vi "Actor Core.vi"(0 "Module in":refnum<class "Module.lvclass">, 11 "Error in":errorcluster caption="Error in (no error)") -> (4 "Module out":refnum<class "Module.lvclass">, 15 "Error out":errorcluster)   [LabVIEW 2019, in "GP Module.lvlib" / "Module.lvclass"]
doc: "GPower Actor Core VI.\n\nSteen Schmidt\nGPower\n9/9 2018"
uses:
  Module.lvclass
  C:/Program Files (x86)/National Instruments/LabVIEW 2019/vi.lib/GPower/Actor/Library/Actor Class/Actor.lvclass
  Module.lvclass/Module.ctl
  <vilib>/GPower/Actor/Library/Actor Class/Actor.lvclass/Actor.ctl
  <vilib>/GPower/Actor/Library/Actor Interface Class/Actor Interface.lvclass/Actor Interface.ctl
  <vilib>/GPower/Message/Library/Message Class/Message.lvclass/Message.ctl
  <vilib>/GPower/Logger/Library/Logger Class/Logger.lvclass/Logger.ctl
  <vilib>/GPower/Actor/Library/Actor Interface Class/Accessors/Get Actor Name.vi
  <vilib>/GPower/Logger/Library/Logger Class/Logger/Log.vi
  <vilib>/GPower/Message/Library/Message Class/Accessors/Get Name.vi
  <vilib>/GPower/Error/Library/ErrorType.vi
  <vilib>/GPower/Logger/Library/Logger Class/Accessors/Get Enabled State.vi
  <vilib>/GPower/Logger/Library/Logger Class/Accessors/Get Severity Level Threshold.vi
  <vilib>/GPower/Logger/Library/Logger Class/Logger/Promote.vi
  <vilib>/GPower/Error/Library/SplitAppended.vi
  <vilib>/GPower/Logger/Library/Logger Class/Accessors/Get Error And Warning Promotion.vi
  <vilib>/GPower/Error/Library/SubVIs/ExplanationToError.vi
  <vilib>/dlg_ctls.llb/Space Constant.vi
  <vilib>/Utility/error.llb/Trim Whitespace.vi
  <vilib>/Utility/error.llb/Error Code Database.vi
  <vilib>/GPower/Error/Library/SubVIs/SetStatus.vi
  <vilib>/GPower/Error/Library/AppendErrors.vi
  <vilib>/GPower/Error/Library/Append/AppendSingle.vi
  <vilib>/GPower/Logger/Library/Logger Class/Logger.lvclass
  <vilib>/GPower/Actor/Library/Actor Class/Actor.lvclass
  <vilib>/GPower/Actor/Library/Responder Class/Responder.lvclass
panel:
  in  "Stop":bool
  out "Boolean":bool
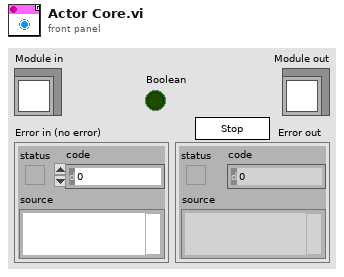
[diagram p1: front panel]
types:
  T1 = typedef "GP Actor.lvlib/Actor Interface.lvclass/Registered Actor Events.ctl" = cluster{"Actor Messages":refnum<event-registration>, "Actor Stopped":refnum<event-registration>, "Actor Stop":refnum<event-registration>}
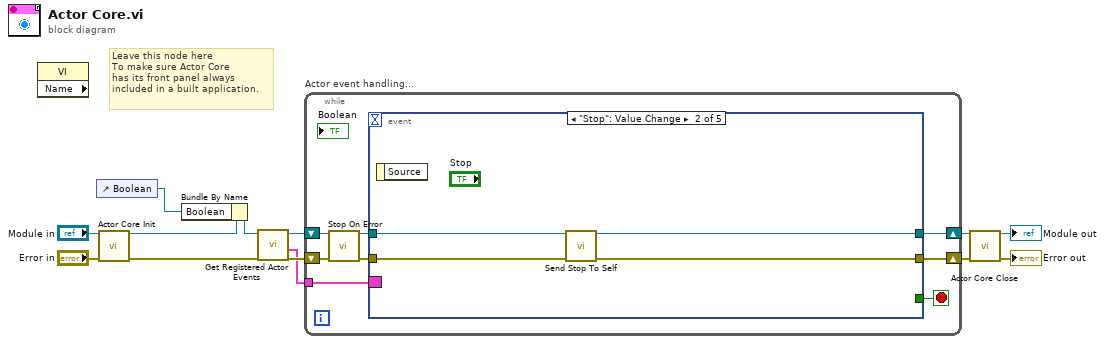
[diagram p0: block diagram]
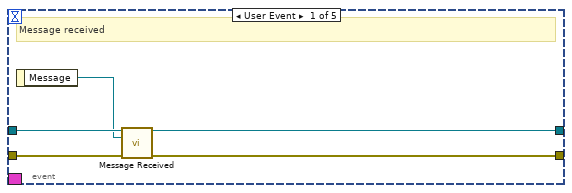
[diagram p2: hidden frame]
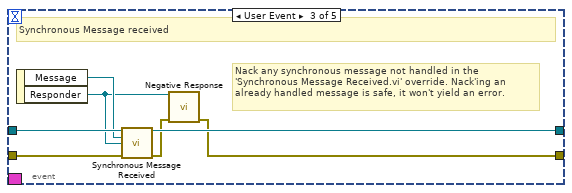
[diagram p3: hidden frame]
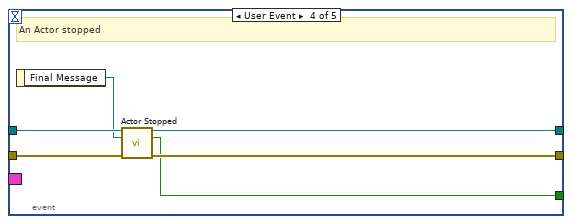
[diagram p4: hidden frame]
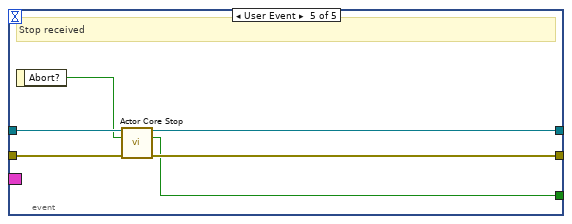
[diagram p5: hidden frame]
diagram:
  # "Leave this node here\nTo make sure Actor Core\nhas its front panel always\nincluded in a built application."
  n1 = property class="VI" props=["Name"]() -> ()  [unwired: 2 in, 3 out]
  n2 = control-ref of="Boolean"() -> (w1:refnum<vi>)
  n3 = call <vilib>:"Actor Core Init.vi"("Actor in"="Module in", "Error in"="Error in") -> ("Actor out"=w3:refnum<class "Module.lvclass">, "Error out"=w10:errorcluster)  [unwired: 12 in]
  n4 = Bundle By Name(cluster=w3, "Boolean"=w1) -> (w2:refnum<class "Module.lvclass">)
  n5 = call <vilib>:"Get Registered Actor Events.vi"("Actor in"=w2) -> ("Registered Actor Events"=w4:T1, "Actor out"=w5:refnum<class "Module.lvclass">)  [unwired: 9 in]
  n6 = while "Actor event handling..." {
    tunnel: w4 -> [w13]
    shift-right: [w19] -> w9
    shift-left: w10 -> [w15]
    shift-right: [w18] -> w8
    shift-left: w5 -> [w17]
    stop <- w20 stop-if-true
    n7 = call <vilib>:"Stop On Error.vi"("Actor in"=w17, "Error in"=w15) -> ("Actor out"=w16:refnum<class "Module.lvclass">, "Error out"=w14:errorcluster)  [unwired: 12 in]
    n8 = event shown="[1] \"Stop\": Value Change" {
      selector: w13 -> [_ _ _ _ _]
      dyn-events: _ -> [_ _ _ _ _]
      timeout: _ -> [_ _ _ _ _]
      tunnel: w16 -> [w25 w28 w34 w41 w48]
      tunnel: w14 -> [w23 w29 w36 w42 w46]
      tunnel: [w22 w26 w31 w40 w45] -> w19
      tunnel: [w24 w27 w35 w39 w47] -> w18
      tunnel: [_ _ _ w37 w44] -> w20
      event User Event {
        # "Message received"
        n9 = event-data() -> ("Message"=w21:refnum<class "Message.lvclass">)  [unwired: 1 in]
        n10 = call <vilib>:"Message Received.vi"("Actor in"=w25, "Message"=w21, "Error in"=w23) -> ("Actor out"=w24:refnum<class "Module.lvclass">, "Error out"=w22:errorcluster)  [unwired: 11 in]
      }
      event "Stop": Value Change {
        n11 = event-data() -> ()  [unwired: 1 in, 1 out]
        n12 = call <vilib>:"Send Stop To Self.vi"("Self in"=w28, "error in (no error)"=w29) -> ("Self out"=w27:refnum<class "Module.lvclass">, "error out"=w26:errorcluster)  [unwired: 12 in]
      }
      event User Event {
        # "Nack any synchronous message not handled in the 'Synchronous Message Received.vi' override. Nack'ing an already handled message is safe, it won't yield an error."
        # "Synchronous Message received"
        n13 = event-data() -> ("Message"=w33:refnum<class "Message.lvclass">, "Responder"=w30:refnum<class "Responder.lvclass">)  [unwired: 1 in]
        n14 = call <vilib>:"Synchronous Message Received.vi"("Actor in"=w34, "Message"=w33, "Responder"=w30, "Error in"=w36) -> ("Actor out"=w35:refnum<class "Module.lvclass">, "Error out"=w32:errorcluster)  [unwired: 10 in]
        n15 = call <vilib>:"Negative Response.vi"("Responder"=w30, "Error in"=w32) -> ("Error out"=w31:errorcluster)  [unwired: 13 in]
      }
      event User Event {
        # "An Actor stopped"
        n16 = event-data() -> ("Final Message"=w38:refnum<class "Final Message.lvclass">)  [unwired: 1 in]
        n17 = call <vilib>:"Actor Stopped.vi"("Actor in"=w41, "Stopped Actor Final Message"=w38, "Error in"=w42) -> ("Actor out"=w39:refnum<class "Module.lvclass">, "Stop Myself Now?"=w37:bool, "Error out"=w40:errorcluster)  [unwired: 10 in]
      }
      event User Event {
        # "Stop received"
        n18 = event-data() -> ("Abort?"=w43:bool)  [unwired: 1 in]
        n19 = call <vilib>:"Actor Core Stop.vi"("Actor in"=w48, "Abort?"=w43, "Error in"=w46) -> ("Actor out"=w47:refnum<class "Module.lvclass">, "Stop Myself Now?"=w44:bool, "Error out"=w45:errorcluster)  [unwired: 10 in]
      }
    }
  }
  n20 = call <vilib>:"Actor Core Close.vi"("Actor in"=w8, "Error in"=w9) -> ("Actor out"=→"Module out":refnum<class "Module.lvclass">, "Error out"=→"Error out":errorcluster)  [unwired: 12 in]
